vi "Configure Range Limits.vi"(7 "Unit Address (1)":u8=1, 8 "error in (no error)":errorcluster, 9 "Range Low (N/A)":i32, 10 "Range High (N/A)":i32, 11 "VISA resource name":refnum<visa-resource-name>) -> (0 "error out":errorcluster, 3 "VISA resource name out":refnum<visa-resource-name>)   [LabVIEW 2014, in "Eurotherm 35xx Series.lvlib"]
doc: "This VI sets the limits (electrical) of input level."
uses:
  <instrlib>/Eurotherm 35xx Series/Eurotherm 35xx Series.lvlib
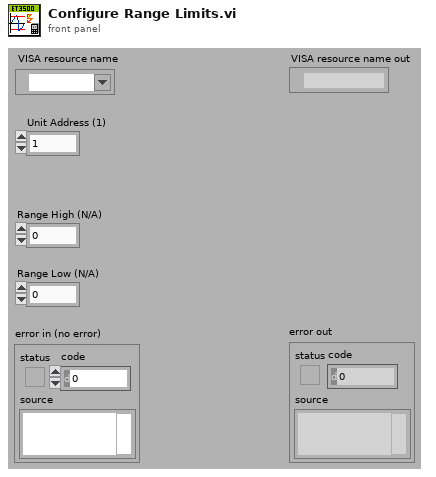
[diagram p1: front panel]
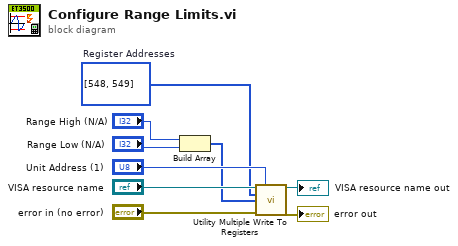
[diagram p0: block diagram]
diagram:
  w4 = i32[] [548, 549]  # Register Addresses
  n1 = Build Array("Range High (N/A)", "Range Low (N/A)") -> (w1:i32[])
  n2 = call <instrlib>:"Utility Multiple Write To Registers.vi"("VISA resource name"="VISA resource name", "Unit Address (1)"="Unit Address (1)", "Registers Addresses (0)"=w4, "Data (0)"=w1, "error in (no error)"="error in (no error)") -> ("VISA resource name out"=→"VISA resource name out":refnum<visa-resource-name>, "error out"=→"error out":errorcluster)  [unwired: 9 in]
